vi "setChanged.vi"(8 "error in (no error)":errorcluster, 10 "Changed?":bool, 11 "WeatherData in":refnum<class "WeatherData.lvclass">) -> (0 "error out":errorcluster, 3 "WeatherData out":refnum<class "WeatherData.lvclass">)   [LabVIEW 2017, in "WeatherData.lvclass"]
uses:
  WeatherData.lvclass
  WeatherData.lvclass/WeatherData.ctl
  Observer/Observer.lvclass
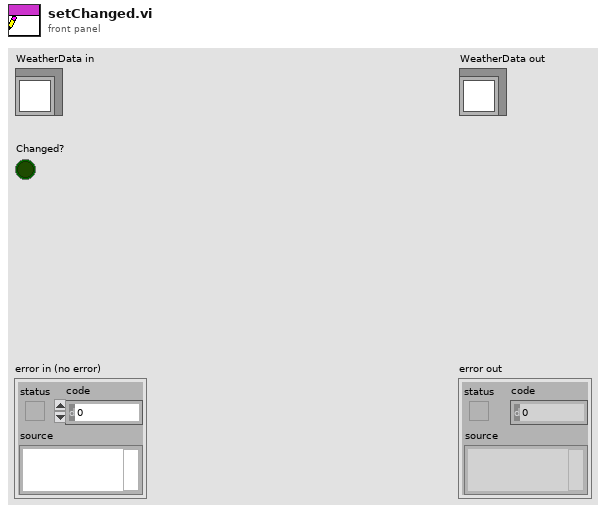
[diagram p1: front panel]
types:
  T1 = cluster{"Temperature":dbl, "Humidity":dbl, "Pressure":dbl}
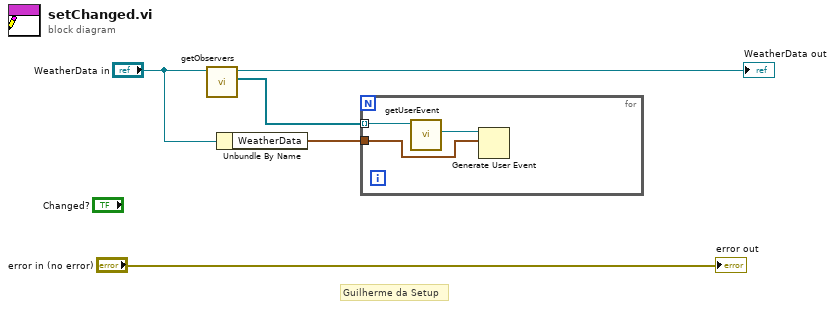
[diagram p0: block diagram]
diagram:
  # "Guilherme da Setup"
  n1 = call-dynamic "getObservers.vi"("WeatherData in"="WeatherData in") -> ("Observers"=w3:refnum<class "Observer.lvclass">[], "WeatherData out"=→"WeatherData out":refnum<class "WeatherData.lvclass">)  [unwired: 8 in, 1 out]
  n2 = Unbundle By Name("WeatherData in") -> ("WeatherData"=w4:T1)
  n3 = for {
    tunnel: w3 -> [w8] mode=indexing
    tunnel: w4 -> [w6]
    n4 = call-dynamic "getUserEvent.vi"("Observer in"=w8) -> ("user event"=w7:refnum<user-event>)  [unwired: 8 in, 2 out]
    n5 = Generate User Event(user event=w7, event data cluster=w6) -> ()  [unwired: 2 in, 2 out]
  }
  "error out" <- "error in (no error)"
